vi "server.vi"() -> ()   [LabVIEW 2018]
panel:
  in  "待发送字符串":string
  in  "端口号":i32
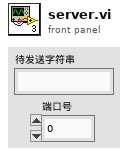
[diagram p1: front panel]
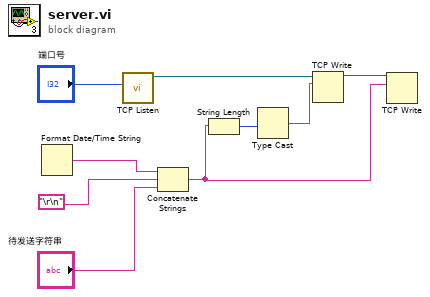
[diagram p0: block diagram]
diagram:
  n1 = Format Date/Time String() -> (date/time string=w7:string)  [unwired: 3 in]
  n2 = call <vilib>:"TCP Listen.vi"("port"="端口号") -> ("connection ID"=w8:refnum<k5>)  [unwired: 6 in, 4 out]
  n3 = Concatenate Strings(w7, "\r\n", "待发送字符串") -> (w1:string)
  n4 = String Length(string=w1) -> (length=w4:i32)
  n5 = Type Cast(x=w4) -> (*(type *) &x=w3:string)  [unwired: 1 in]
  n6 = TCP Write(connection ID=w8, data in=w3) -> (connection ID out=w2:refnum<k5>)  [unwired: 2 in, 2 out]
  n7 = TCP Write(connection ID=w2, data in=w1) -> ()  [unwired: 2 in, 3 out]
